vi "Binary Bad Tube Search SubVI.vi"(5 "End Tube Number":i32, 7 "Beginning Tube Number":i32, 8 "Clear Pin Task In":refnum<k21>, 9 "Write Pin Task In":refnum<k21>, 10 "Sync Pin Task In":refnum<k21>, 11 "Data Pin Task In":refnum<k21>) -> (0 "Clear Pin Task Out":refnum<k21>, 1 "Write Pin Task Out":refnum<k21>, 2 "Sync Pin Task Out":refnum<k21>, 3 "Data Pin Task Out":refnum<k21>)   [LabVIEW 2020]
uses:
  <vilib>/numeric/Random Number (Range) DBL.vi
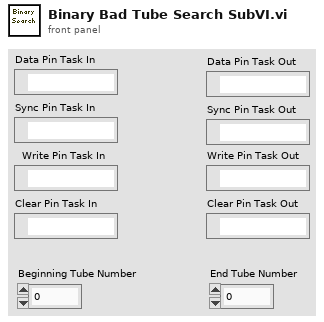
[diagram p1: front panel]
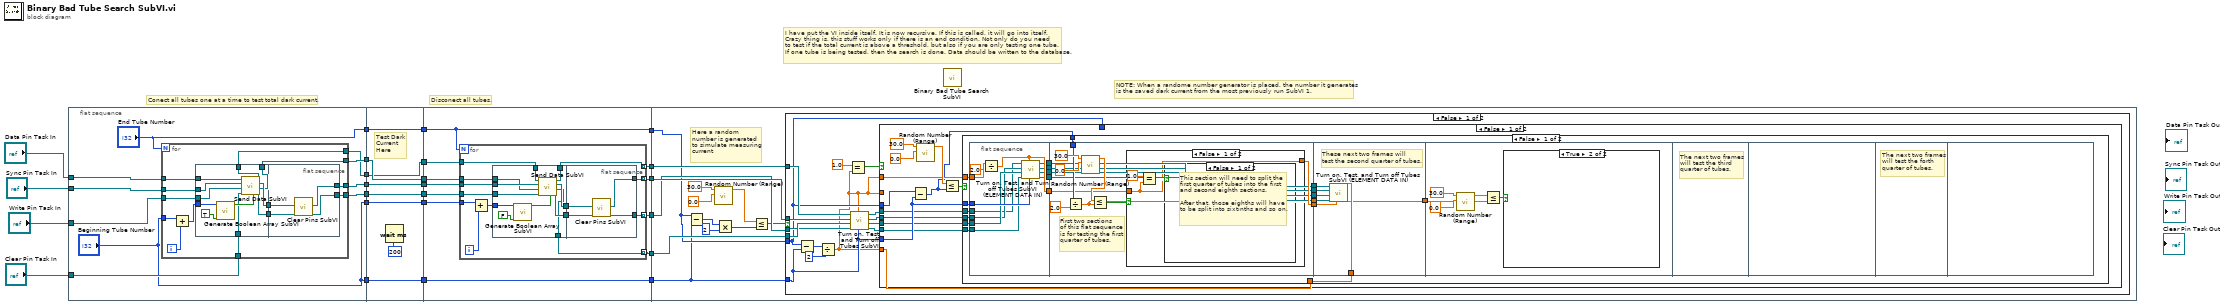
[diagram p0: block diagram]
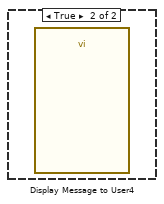
[diagram p2: hidden frame]
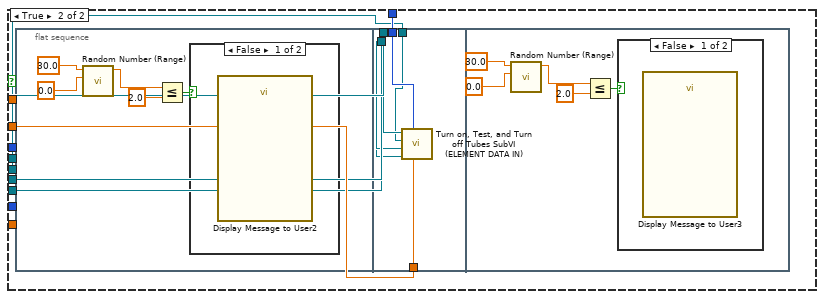
[diagram p6: hidden frame]
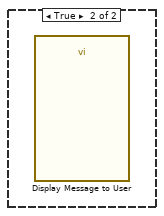
[diagram p9: hidden frame]
diagram:
  # "NOTE: When a randome number generator is placed, the number it generates\nis the saved dark current from the most previously run SubVI 1."
  # "I have put the VI inside itself. It is now recursive. If this is called, it will go into itself.\nCrazy thing is, this stuff works only if there is an end condition. Not only do you need\nto test if the total current is above a threshold, but also if you are only testing one tube.\nIf one tube is being tested, then the search is done. Data should be written to the database."
  # "Disconect all tubes."
  # "Conect all tubes one at a time to test total dark current."
  n1 = flat-sequence {
    tunnel: "Data Pin Task In" -> [w34]
    tunnel: "Sync Pin Task In" -> [w33]
    tunnel: "Write Pin Task In" -> [w32]
    tunnel: "Clear Pin Task In" -> [w31]
    tunnel: ["End Tube Number"] -> w19
    tunnel: [w29] -> w17
    tunnel: [w28] -> w15
    tunnel: [w27] -> w13
    tunnel: [w26] -> w11
    tunnel: ["Beginning Tube Number"] -> w8
    tunnel: ["Beginning Tube Number"] -> w5
    tunnel: [w69] -> w20
    tunnel: w19 -> [w69]
    tunnel: [w68] -> w18
    tunnel: w17 -> [w68]
    tunnel: [w67] -> w16
    tunnel: w15 -> [w67]
    tunnel: [w66] -> w14
    tunnel: w13 -> [w66]
    tunnel: [w65] -> w12
    tunnel: w11 -> [w65]
    tunnel: [w64] -> w9
    tunnel: w8 -> [w64]
    tunnel: [w63] -> w6
    tunnel: w5 -> [w63]
    tunnel: w20 -> [w77]
    tunnel: w18 -> [w81]
    tunnel: w16 -> [w80]
    tunnel: w14 -> [w79]
    tunnel: w12 -> [w78]
    tunnel: [w77] -> w10
    tunnel: w9 -> [w76]
    tunnel: [w75] -> w7
    tunnel: w6 -> [w75]
    tunnel: [w74] -> w4
    tunnel: [w73] -> w3
    tunnel: [w72] -> w2
    tunnel: [w71] -> w1
    tunnel: w10 -> [w111]
    tunnel: w7 -> [w110]
    tunnel: w4 -> [w119]
    tunnel: w3 -> [w118]
    tunnel: w2 -> [w117]
    tunnel: w1 -> [w116]
    frame #0 {
      n2 = for {
        N: "End Tube Number" -> [_]
        tunnel: w34 -> [w47]
        tunnel: w33 -> [w46]
        tunnel: w32 -> [w45]
        tunnel: w31 -> [w44]
        tunnel: [w41] -> w29
        tunnel: [w40] -> w28
        tunnel: [w39] -> w27
        tunnel: [w38] -> w26
        tunnel: "Beginning Tube Number" -> [w35]
        i -> [w36]
        n3 = Add(x=w35, y=w36) -> (x+y=w37:i32)
        n4 = flat-sequence {
          tunnel: w37 -> [w56]
          tunnel: w47 -> [w55]
          tunnel: w46 -> [w54]
          tunnel: w45 -> [w53]
          tunnel: w44 -> [w52]
          tunnel: [w51] -> w43
          tunnel: [w50] -> w42
          tunnel: [w49] -> w39
          tunnel: [w48] -> w38
          tunnel: w43 -> [w62]
          tunnel: w42 -> [w61]
          tunnel: [w60] -> w41
          tunnel: [w59] -> w40
          frame #0 {
            n5 = call "Generate Boolean Array SubVI.vi"("Activate: 1\nDeactivate: 0"=TRUE, "Tube"=w56) -> ("Boolean array"=w57:bool[])  [unwired: 9 in]
            n6 = call "Send Data SubVI.vi"("Data Pin Task In"=w55, "Sync Pin Task In"=w54, "Write Pin Task In"=w53, "Clear Pin Task In"=w52, "Data"=w57) -> ("Data Pin Task Out"=w48:refnum<k21>, "Sync Pin Task Out"=w51:refnum<k21>, "Write Pin Task Out"=w49:refnum<k21>, "Clear Pin Task Out"=w50:refnum<k21>)  [unwired: 1 in]
          }
          frame #1 {
            n7 = call "Clear Pins SubVI.vi"("Clear Pin Task In"=w61, "Sync Pin Task In"=w62) -> ("Clear Pin Task Out"=w59:refnum<k21>, "Sync Pin Task Out"=w60:refnum<k21>)  [unwired: 8 in]
          }
        }
      }
    }
    frame #1 {
      # "Test Dark \nCurrent \nHere"
      n8 = Wait (ms)(milliseconds to wait=u32 200) -> ()  [unwired: 1 out]
    }
    frame #2 {
      n9 = for {
        N: w77 -> [_]
        tunnel: w81 -> [w92]
        tunnel: w80 -> [w91]
        tunnel: w79 -> [w90]
        tunnel: w78 -> [w89]
        tunnel: w76 -> [w86]
        tunnel: [w85] -> w74 mode=indexing
        tunnel: [w84] -> w73 mode=indexing
        tunnel: [w83] -> w72 mode=indexing
        tunnel: [w82] -> w71 mode=indexing
        i -> [w87]
        n10 = Add(x=w86, y=w87) -> (x+y=w88:i32)
        n11 = flat-sequence {
          tunnel: w88 -> [w103]
          tunnel: [w102] -> w94
          tunnel: [w101] -> w93
          tunnel: w92 -> [w100]
          tunnel: w91 -> [w99]
          tunnel: w90 -> [w98]
          tunnel: w89 -> [w97]
          tunnel: [w96] -> w85
          tunnel: [w95] -> w83
          tunnel: w94 -> [w109]
          tunnel: w93 -> [w108]
          tunnel: [w107] -> w84
          tunnel: [w106] -> w82
          frame #0 {
            n12 = call "Generate Boolean Array SubVI.vi"("Activate: 1\nDeactivate: 0"=FALSE, "Tube"=w103) -> ("Boolean array"=w104:bool[])  [unwired: 9 in]
            n13 = call "Send Data SubVI.vi"("Data Pin Task In"=w97, "Sync Pin Task In"=w100, "Write Pin Task In"=w98, "Clear Pin Task In"=w99, "Data"=w104) -> ("Data Pin Task Out"=w96:refnum<k21>, "Sync Pin Task Out"=w102:refnum<k21>, "Write Pin Task Out"=w95:refnum<k21>, "Clear Pin Task Out"=w101:refnum<k21>)  [unwired: 1 in]
          }
          frame #1 {
            n14 = call "Clear Pins SubVI.vi"("Clear Pin Task In"=w108, "Sync Pin Task In"=w109) -> ("Clear Pin Task Out"=w106:refnum<k21>, "Sync Pin Task Out"=w107:refnum<k21>)  [unwired: 8 in]
          }
        }
      }
    }
    frame #3 {
      # "Here a random\nnumber is generated\nto simulate measuring\ncurrent"
      n15 = Subtract(x=w111, y=w110) -> (x-y=w112:i32)
      n16 = call-poly <vilib>:"Random Number (Range).vi"("lower bound (0)"=0.0, "upper bound (100)"=30.0) -> ("number"=w115:dbl)  [unwired: 9 in]
      n17 = Multiply(x=w112, y=2) -> (x*y=w114:i32)
      n18 = Less Or Equal?(x=w115, y=w114) -> (x <= y?=w113:bool)
      n19 = case shown="False" w113 {
        tunnel: w111 -> [w125 _]
        tunnel: w110 -> [w124 _]
        tunnel: w119 -> [w135 _]
        tunnel: w118 -> [w134 _]
        tunnel: w117 -> [w133 _]
        tunnel: w116 -> [w132 _]
        frame False {
          n20 = Subtract(x=w125, y=w124) -> (x-y=w137:i32)
          n21 = Divide(x=w137, y=2) -> (x/y=w123:dbl)
          n22 = Equal?(x=1.0, y=w123) -> (x = y?=w130:bool)
          n23 = call "Turn on, Test, and Turn off Tubes SubVI.vi"("Begin Tube #"=w124, "End Tube #"=w123, "Clear Pin in"=w132, "Write Pin in"=w133, "Sync Pin in"=w134, "Data Pin in"=w135) -> ("Clear Pin out"=w126:refnum<k21>, "Write Pin out"=w127:refnum<k21>, "Sync Pin out"=w128:refnum<k21>, "Data Pin out"=w129:refnum<k21>)  [unwired: 2 in]
          n24 = case shown="False" w130 {
            tunnel: w123 -> [_ w216]
            tunnel: w125 -> [_ w215]
            tunnel: w129 -> [w140 w214]
            tunnel: w128 -> [w141 w213]
            tunnel: w127 -> [w142 w212]
            tunnel: w126 -> [w143 w211]
            tunnel: w125 -> [w148 _]
            tunnel: w124 -> [w144 _]
            tunnel: w123 -> [w145 _]
            tunnel: w123 -> [w138 _]
            frame False {
              n25 = Subtract(x=w148, y=w144) -> (x-y=w139:i32)
              n26 = call-poly <vilib>:"Random Number (Range).vi"("lower bound (0)"=0.0, "upper bound (100)"=30.0) -> ("number"=w147:dbl)  [unwired: 9 in]
              n27 = Less Or Equal?(x=w147, y=w139) -> (x <= y?=w146:bool)
              n28 = case shown="False" w146 {
                tunnel: w145 -> [w170 _]
                tunnel: w144 -> [w169 _]
                tunnel: w143 -> [w168 _]
                tunnel: w142 -> [w167 _]
                tunnel: w141 -> [w166 _]
                tunnel: w140 -> [w165 _]
                tunnel: w139 -> [w164 _]
                tunnel: w138 -> [w161 _]
                frame False {
                  n29 = flat-sequence {
                    tunnel: w170 -> [w182]
                    tunnel: w169 -> [w180]
                    tunnel: w168 -> [w179]
                    tunnel: w167 -> [w178]
                    tunnel: w166 -> [w177]
                    tunnel: w165 -> [w176]
                    tunnel: [w175] -> w163
                    tunnel: [w174] -> w159
                    tunnel: [w173] -> w157
                    tunnel: [w172] -> w155
                    tunnel: [w171] -> w153
                    tunnel: w164 -> [w191]
                    tunnel: w163 -> [w189]
                    tunnel: [w188] -> w162
                    tunnel: [w187] -> w160
                    tunnel: w159 -> [w187]
                    tunnel: [w186] -> w158
                    tunnel: w157 -> [w186]
                    tunnel: [w185] -> w156
                    tunnel: w155 -> [w185]
                    tunnel: [w184] -> w154
                    tunnel: w153 -> [w184]
                    tunnel: [w183] -> w151
                    tunnel: w162 -> [w205]
                    tunnel: w161 -> [w204]
                    tunnel: w160 -> [w203]
                    tunnel: w158 -> [w202]
                    tunnel: w156 -> [w201]
                    tunnel: w154 -> [w200]
                    tunnel: [w199] -> w152
                    tunnel: w151 -> [w199]
                    tunnel: w152 -> [w207]
                    frame #0 {
                      n30 = Divide(x=w182, y=2.0) -> (x/y=w175:dbl)
                      n31 = call "Turn on, Test, and Turn off Tubes SubVI (ELEMENT DATA IN).vi"("Begin Tube #"=w180, "End Tube #"=w175, "Clear Pin in"=w179, "Write Pin in"=w178, "Sync Pin in"=w177, "Data Pin in"=w176) -> ("Clear Pin out"=w171:refnum<k21>, "Write Pin out"=w172:refnum<k21>, "Sync Pin out"=w173:refnum<k21>, "Data Pin out"=w174:refnum<k21>)  [unwired: 2 in]
                    }
                    frame #1 {
                      # "First two sections\nof this flat sequence\nis for testing the first\nquarter of tubes."
                      n32 = Divide(x=w191, y=2.0) -> (x/y=w183:dbl)
                      n33 = call-poly <vilib>:"Random Number (Range).vi"("lower bound (0)"=0.0, "upper bound (100)"=30.0) -> ("number"=w193:dbl)  [unwired: 9 in]
                      n34 = Less Or Equal?(x=w193, y=w183) -> (x <= y?=w190:bool)
                      n35 = case shown="False" w190 {
                        tunnel: w189 -> [w196 _]
                        tunnel: [w196 _] -> w188
                        frame False {
                          n36 = Equal?(x=1.0, y=w196) -> (x = y?=w197:bool)
                          n37 = case shown="False" w197 {
                            frame False {
                              # "This section will need to split the \nfirst quarter of tubes into the first \nand second eighth sections.\n\nAfter that, those eighths will have \nto be split into sixtinths and so on."
                            }
                            frame True {
                              n38 = call "Display Message to User4"() -> ()  [unwired: 10 in, 2 out]
                            }
                          }
                        }
                        frame True {
                        }
                      }
                    }
                    frame #2 {
                      # "These next two frames will\ntest the second quarter of tubes."
                      n39 = call "Turn on, Test, and Turn off Tubes SubVI (ELEMENT DATA IN).vi"("Begin Tube #"=w205, "End Tube #"=w204, "Clear Pin in"=w200, "Write Pin in"=w201, "Sync Pin in"=w202, "Data Pin in"=w203) -> ()  [unwired: 2 in, 4 out]
                    }
                    frame #3 {
                      n40 = call-poly <vilib>:"Random Number (Range).vi"("lower bound (0)"=0.0, "upper bound (100)"=30.0) -> ("number"=w208:dbl)  [unwired: 9 in]
                      n41 = Less Or Equal?(x=w208, y=w207) -> (x <= y?=w206:bool)
                      n42 = case shown="True" w206 {
                        frame False {
                        }
                        frame True {
                        }
                      }
                    }
                    frame #4 {
                      # "The next two frames\nwill test the third \nquarter of tubes."
                    }
                    frame #5 {
                    }
                    frame #6 {
                      # "The next two frames\nwill test the forth\nquarter of tubes."
                    }
                    frame #7 {
                    }
                  }
                }
                frame True {
                }
              }
            }
            frame True {
              n43 = flat-sequence {
                tunnel: w216 -> [w226]
                tunnel: w215 -> [w227]
                tunnel: w214 -> [w225]
                tunnel: w213 -> [w224]
                tunnel: w212 -> [w223]
                tunnel: w211 -> [w222]
                frame #0 {
                  n44 = call-poly <vilib>:"Random Number (Range).vi"("lower bound (0)"=0.0, "upper bound (100)"=30.0) -> ("number"=w219:dbl)  [unwired: 9 in]
                  n45 = Less Or Equal?(x=w219, y=2.0) -> (x <= y?=w217:bool)
                  n46 = case shown="False" w217 {
                    frame False {
                      n47 = call "Display Message to User2"() -> ()  [unwired: 10 in, 2 out]
                    }
                    frame True {
                    }
                  }
                }
                frame #1 {
                  n48 = call "Turn on, Test, and Turn off Tubes SubVI (ELEMENT DATA IN).vi"("Begin Tube #"=w226, "End Tube #"=w227, "Clear Pin in"=w222, "Write Pin in"=w223, "Sync Pin in"=w224, "Data Pin in"=w225) -> ()  [unwired: 2 in, 4 out]
                }
                frame #2 {
                  n49 = call-poly <vilib>:"Random Number (Range).vi"("lower bound (0)"=0.0, "upper bound (100)"=30.0) -> ("number"=w230:dbl)  [unwired: 9 in]
                  n50 = Less Or Equal?(x=w230, y=2.0) -> (x <= y?=w228:bool)
                  n51 = case shown="False" w228 {
                    frame False {
                      n52 = call "Display Message to User3"() -> ()  [unwired: 10 in, 2 out]
                    }
                    frame True {
                    }
                  }
                }
              }
            }
          }
        }
        frame True {
          n53 = call "Display Message to User"() -> ()  [unwired: 10 in, 2 out]
        }
      }
    }
  }
  n54 = call "Binary Bad Tube Search SubVI.vi"() -> ()  [unwired: 8 in, 4 out]
